vi "AlazarReadBuffer.vi"(7 "Digitizer Settings":T1={"Digitizer delay (us) "=18.666667, "rf points per line"=4000, "lines per plane"=139, "Samp Rate (Hz)"=100000000.0, "Additional dig delay (us)"=0.0, "Voltage Scale"=0.4, "Pre-Looks"=0, "Offset delay (us)"=2.0, "bits A/D"=0, "Avg Num"=1, "DigTimeOut"=5.0, "Rel Dig Delay"=0.0, "Dig Ch"=0, "LeCroyCluster"={"LeCroy Channels"=[TRUE, FALSE, FALSE, FALSE], "LC read pt offset"=0.0, "Sweep Avg"=FALSE}, "Main Digitizer"=enum."NI Digitizer", "Dig Config"=enum."Single channel", "Digitizer ID Cluster"={"Acqiris/Alazar/SP ID"=[], "NI Instr Handles"=[], "LeCroy VISA"="", "GaGe Handle"={"Handle"=0, "Sample size"=0, "Resolution"=0, "Offset"=0, "Channels"=0, "Boards"=0}, "ATS Ref"="ATS9350", "Acqiris Address"=["PCI::INSTR0"], "ADQRef"=refnum, "adq_cu_ptr"=refnum}, "Trigger Settings"={"Trig Source"=1, "Trig Coupling"=0, "Trig Slope"=0, "Level (mV)"=1500.0}, "Bulk Acq"=FALSE, "Bulk Start Indexes"=[], "Data Ref RF"=refnum, "NI ID/Channel"=[], "Total Dig CH"=1, "Xtra Ann Trig delay (us)"=10.0, "Fix Z Delay?"=FALSE, "One Way Transmission?"=FALSE, "Data Ref Log"=refnum} {"Trigger Settings"."Trig Slope" items=["Positive", "Negative"]; "Trigger Settings"."Level (mV)" format="%.2f"; "Trigger Settings"."Trig Coupling" items=["DC 1 MOhm", "AC 1 MOhm", "DC 50 Ohm", "AC 50 Ohm"]; "Trigger Settings"."Trig Source" items=["Chan 1", "External"]; "Rel Dig Delay" format="%.2f"; "DigTimeOut" format="%.2f"; "Avg Num" min=1; "Offset delay (us)" format="%.2f"; "Additional dig delay (us)" format="%.2f"; "Digitizer delay (us)" format="%.2f"}, 8 "Extra Shift":u16, 10 "time out":dbl=250.0, 11 "AlazarCluster":T5) -> (0 "Return Code":u32, 1 "Voltage Scale":dbl, 2 "Data Array":i16[](array[numeric]))   [LabVIEW 2022 SP3]
uses:
  -DigitizerRoutines/DigitizerSettings.ctl
  -DigitizerRoutines/DigitizerID.ctl
  -DigitizerRoutines/Digitizer.ctl
  -DigitizerRoutines/DigConfig.ctl
  C:/Windows/System32/ADQAPI_dotNet_helper.dll
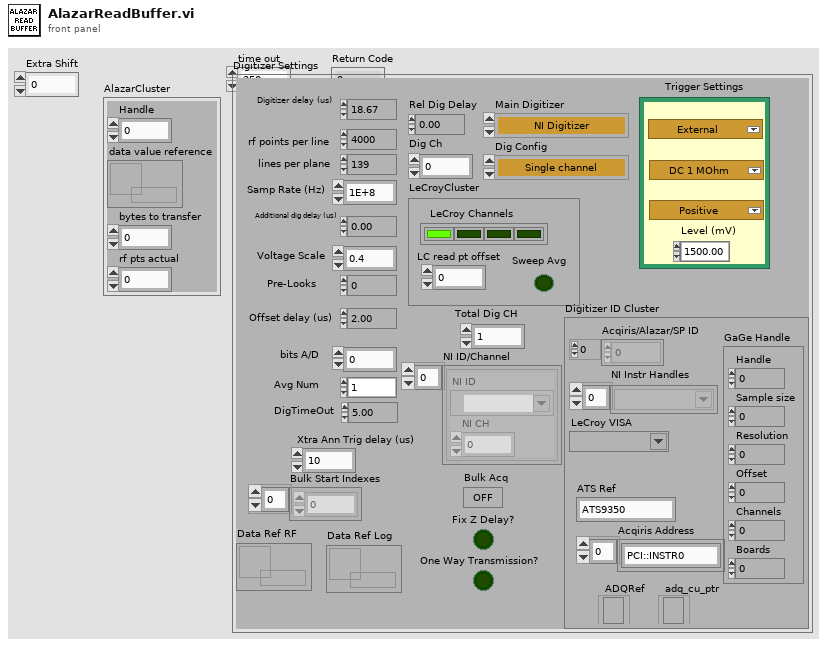
[diagram p1: front panel]
types:
  T1 = typedef "DigitizerSettings.ctl" = cluster{"Digitizer delay (us) ":dbl, "rf points per line":i32, "lines per plane":i32, "Samp Rate (Hz)":dbl, "Additional dig delay (us)":dbl, "Voltage Scale":dbl, "Pre-Looks":i32, "Offset delay (us)":dbl, "bits A/D":i8, "Avg Num":i32, "DigTimeOut":sgl, "Rel Dig Delay":sgl, "Dig Ch":i32, "LeCroyCluster":cluster{"LeCroy Channels":bool[], "LC read pt offset":dbl, "Sweep Avg":bool}, "Main Digitizer":T2, "Dig Config":T3, "Digitizer ID Cluster":T4, "Trigger Settings":cluster{"Trig Source":u16, "Trig Coupling":u16, "Trig Slope":u16, "Level (mV)":dbl}, "Bulk Acq":bool, "Bulk Start Indexes":i32[], "Data Ref RF":refnum<data-value>, "NI ID/Channel":cluster{"NI ID":refnum<k15>, "NI CH":i32}[], "Total Dig CH":i32, "Xtra Ann Trig delay (us)":dbl, "Fix Z Delay?":bool, "One Way Transmission?":bool, "Data Ref Log":refnum<data-value>}
  T2 = typedef "Digitizer.ctl" = enum16{"Acqiris Digitizer", "NI Digitizer", "LeCroy", "GaGe", "AlazarTech", "No Digitizer", "Teledyne"}
  T3 = typedef "DigConfig.ctl" = enum16{"Single channel", "2 Chans w/ 2 Acqiris", "2 Chans w/ 1 Acqiris", "5-CH Pulser New", "5-CH pulser w/ ann array", "5-pass style ann array", "Empty"}
  T4 = typedef "DigitizerID.ctl" = cluster{"Acqiris/Alazar/SP ID":u32[], "NI Instr Handles":refnum<k15>[], "LeCroy VISA":refnum<visa-resource-name>, "GaGe Handle":cluster{"Handle":u32, "Sample size":u32, "Resolution":i32, "Offset":i32, "Channels":u32, "Boards":u32}, "ATS Ref":string, "Acqiris Address":string[], "ADQRef":refnum<k24>, "adq_cu_ptr":refnum<k24>}
  T5 = cluster{"Handle":u32, "data value reference":refnum<data-value>, "bytes to transfer":u32, "rf pts actual":u32}
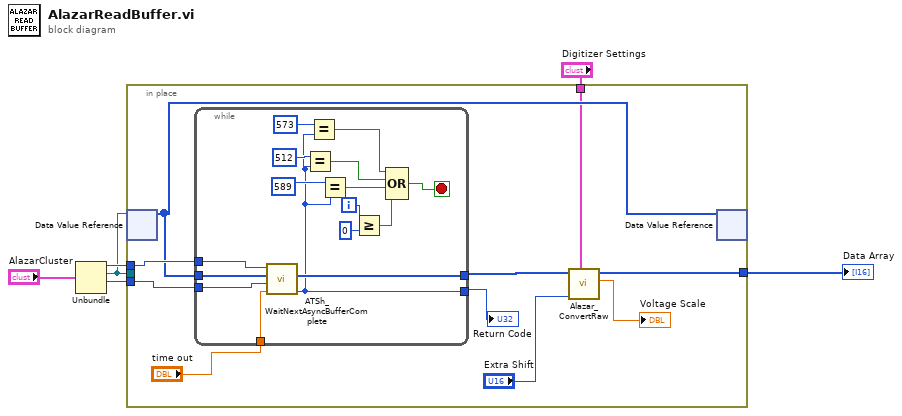
[diagram p0: block diagram]
diagram:
  n1 = Unbundle("AlazarCluster") -> ("Handle"=w5:u32, "data value reference"=w2:refnum<data-value>, "bytes to transfer"=w6:u32)  [unwired: 1 out]
  n2 = in-place {
    in-place-border: w6 -> [w16]
    in-place-border: w5 -> [w15]
    in-place-border: w2 -> [_]
    in-place-border: [w10] -> w3
    in-place-border: "Digitizer Settings" -> [w8]
    n3 = in-place-dvr #1(w2) -> (w9:u16[])  [unwired: 1 out]
    n4 = while {
      tunnel: w15 -> [w32]
      tunnel: "time out" -> [w31]
      tunnel: [w30] -> w13
      tunnel: [w19] -> w14
      tunnel: w9 -> [w26]
      tunnel: w16 -> [w25]
      i -> [w24]
      stop <- w29 stop-if-true
      n5 = call "ATSh_WaitNextAsyncBufferComplete.vi"("uTimeout_ms"=w31, "uBytesPerBuffer"=w25, "pBuffer_In"=w26, "Handle"=w32) -> ("Return Code"=w19:u32, "pBuffer_Out"=w30:u16[])  [unwired: 5 in, 1 out]
      n6 = Equal?(x=u32 512 ("ApiTransferComleted"), y=w19) -> (x = y?=w22:bool)
      n7 = Equal?(x=u32 573, y=w19) -> (x = y?=w17:bool)
      n8 = Equal?(x=u32 589 ("ApiTransferComleted"), y=w19) -> (x = y?=w21:bool)
      n9 = Greater Or Equal?(x=w24, y=0) -> (x >= y?=w20:bool)
      n10 = Compound Arithmetic op=OR(w17, w22, w21, w20) -> (w29:bool)
    }
    "Return Code" <- w14
    n11 = call "Alazar_ConvertRaw.vi"("Digitizer Settings"=w8, "Extra Shift"="Extra Shift", "Buffer"=w13) -> ("Voltage multiplier"=→"Voltage Scale":dbl, "Array"=w10:i16[])  [unwired: 7 in]
    n12 = in-place-dvr #1(w9) -> ()  [unwired: 2 out]
  }
  "Data Array" <- w3
